vi "XboxControllerInput.vi"() -> ()   [LabVIEW 2011]
panel:
  out "x (Rudder)":dbl
  out "y (Prop)":dbl
  in  "stop":bool
  out "Raw Y":i32
  out "Raw X":i32
  out "Propeller Speed":i16(slide) scale=500.0..2500.0
  out "Rudder Pos":i32(slide) scale=500.0..2500.0
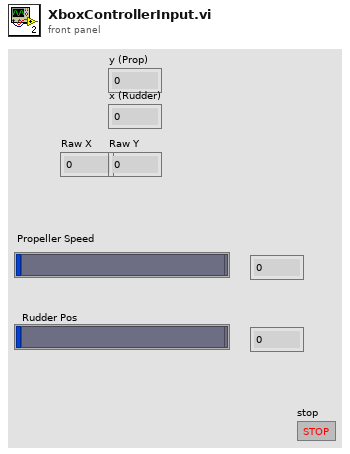
[diagram p1: front panel]
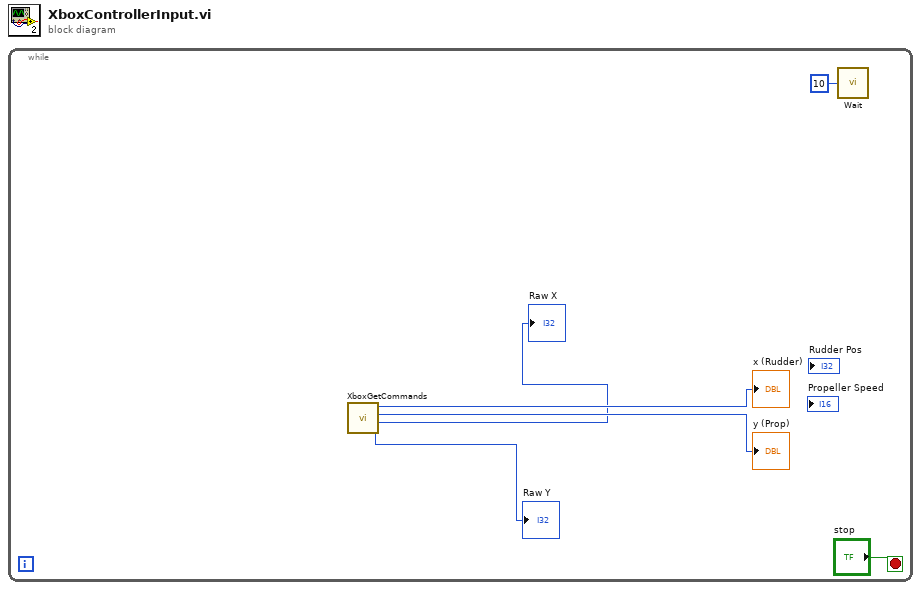
[diagram p0: block diagram]
diagram:
  n1 = while {
    stop <- "stop" stop-if-true
    n2 = call "XboxGetCommands.vi"() -> ("Raw Y"=→"Raw Y":i32, "Raw X"=→"Raw X":i32, "Prop Command"=→"y (Prop)":i8, "Rudder Command"=→"x (Rudder)":i8)  [unwired: 2 in]
    n3 = call "Wait"("Count(mSec)"=u32 10) -> ()  [unwired: 1 out]
  }
